vi "beta_k.vi"(4 "covariance_nontarget":dbl[][](array[numeric]), 6 "covariance_target":dbl[][](array[numeric]), 8 "akl":ext[][](array[numeric]), 9 "u(t+1) = current average":dbl[][](array[numeric]), 11 "T":i64) -> (3 "beta(t)":ext[](array[numeric]))   [LabVIEW 2013]
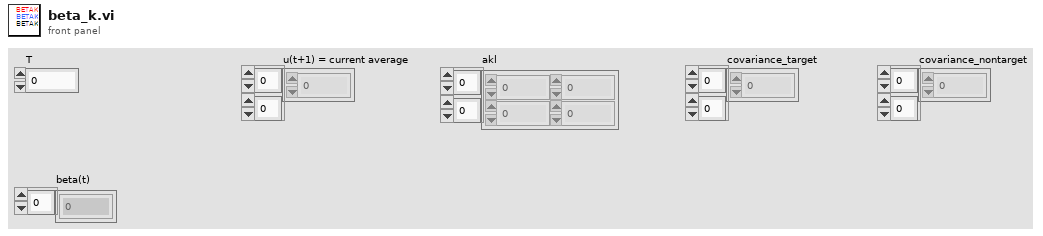
[diagram p1: front panel]
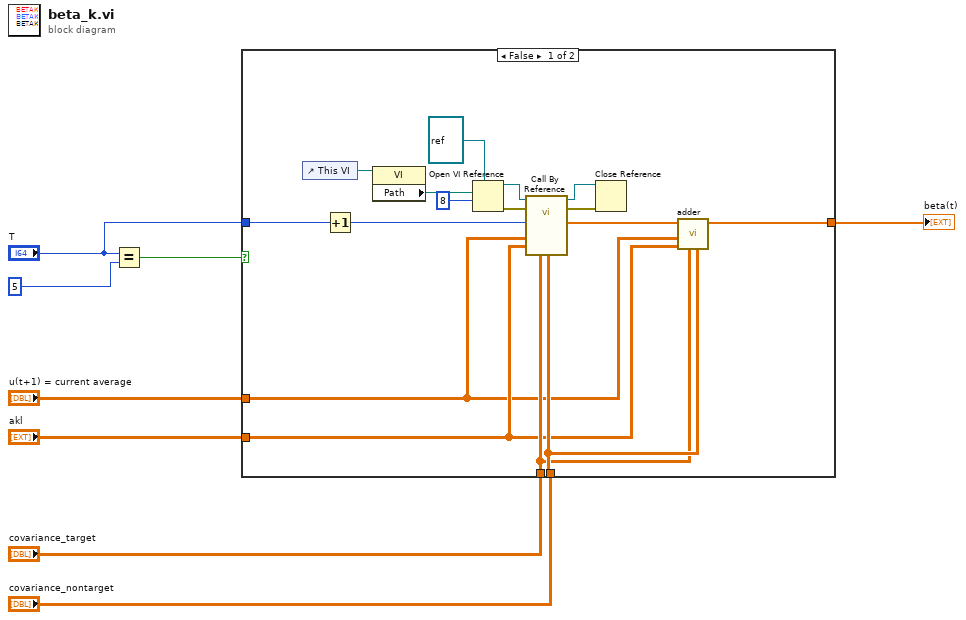
[diagram p0: block diagram]
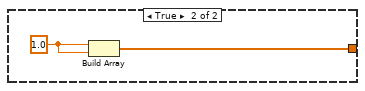
[diagram p2: hidden frame]
diagram:
  n1 = Equal?(x="T", y=i64 5) -> (x = y?=w7:bool)
  n2 = case shown="False" w7 {
    tunnel: "T" -> [w20 _]
    tunnel: "u(t+1) = current average" -> [w9 _]
    tunnel: "akl" -> [w10 _]
    tunnel: [w24 w25] -> w3
    tunnel: "covariance_target" -> [w11 _]
    tunnel: "covariance_nontarget" -> [w12 _]
    frame False {
      n3 = control-ref of="This VI"() -> (w22:refnum<vi>)
      n4 = Increment(x=w20) -> (x+1=w14:i64)
      n5 = property class="VI"(reference=w22) -> ("Path"=w21:path)  [unwired: 1 in, 2 out]
      n6 = Open VI Reference(type specifier VI Refnum (for type only)=refnum<vi> refnum, vi path=w21, options=8) -> (vi reference=w17:refnum<vi>, error out=w18:errorcluster)  [unwired: 3 in]
      n7 = call-by-ref "?"(reference=w17, error in=w18, "covariance_nontarget"=w12, "covariance_target"=w11, "akl"=w10, "u(t+1) = current average"=w9, "T"=w14) -> (reference out=w16:refnum<vi>, error out=w15:errorcluster, "beta(t)"=w13:ext[])  [unwired: 6 in]
      n8 = Close Reference(reference=w16, error in (no error)=w15) -> ()  [unwired: 1 out]
      n9 = call "adder.vi"("covariance_nontarget"=w12, "covariance_target"=w11, "alk"=w10, "u(t+1)"=w9, "beta(t+1)"=w13) -> ("beta(t)"=w24:ext[])  [unwired: 6 in]
    }
    frame True {
      w26 = 1.0 ("element")
      n10 = Build Array(w26, w26) -> (w25:dbl[])
    }
  }
  "beta(t)" <- w3
